vi "数据库访问.vi"() -> ()   [LabVIEW 2018]
uses:
  <vilib>/addons/database/Connection.llb/DB Tools Open Connec (Path).vi
  <vilib>/addons/database/NI_Database_API.lvlib
panel:
  in  "停止":bool
  in  "确定按钮":bool
  out "疫苗数据":T1 {"生产日期" format="%<%Y/%m/%d>T"}
  out "牛奶数据":T2 {"生产日期" format="%<%Y/%m/%d>T"}
  in  "负责人":i32=10003
  in  "牛奶编号":i32=20001
  in  "员工编号":i32=20002
  out "负责人":i32
  out "负责人数据":T3
  out "储运信息":T4 {"记录时间" format="%<%H:%M:%S>T"}
  in  "疫苗编号":i32=10002
  in  "路径":path=path "D:/2019毕业设计/Code/GPData.udl"
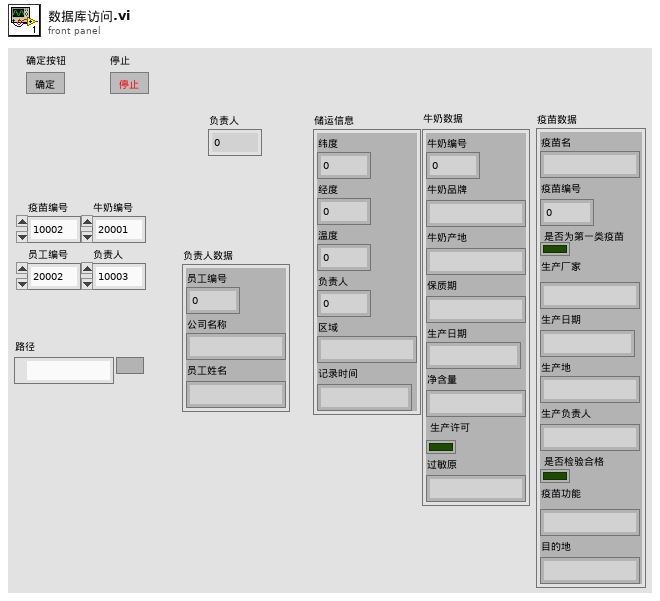
[diagram p1: front panel]
types:
  T1 = typedef "疫苗信息.ctl" = cluster{"疫苗名":string, "疫苗编号":i32, "是否为第一类疫苗":bool, "生产厂家":string, "生产日期":timestamp, "生产地":string, "生产负责人":string, "是否检验合格":bool, "疫苗功能":string, "目的地":string}
  T2 = typedef "牛奶信息.ctl" = cluster{"牛奶编号":i32, "牛奶品牌":string, "牛奶产地":string, "保质期":string, "生产日期":timestamp, "净含量":string, "生产许可":bool, "过敏原":string}
  T3 = typedef "人员信息.ctl" = cluster{"员工编号":i32, "公司名称":string, "员工姓名":string}
  T4 = typedef "储运信息.ctl" = cluster{"纬度":sgl, "经度":sgl, "温度":sgl, "负责人":i32, "区域":string, "记录时间":timestamp}
  T5 = typedef "NI_Database_API.lvlib/Conn ObjectReference.ctl" = refnum<k1>
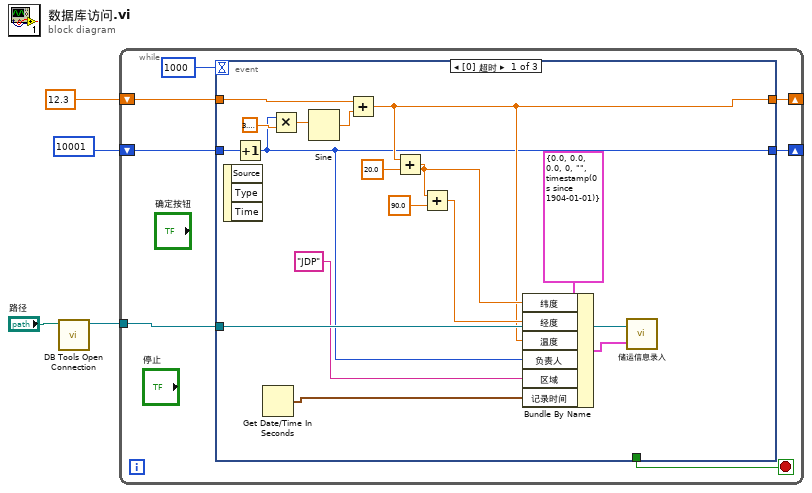
[diagram p0: block diagram]
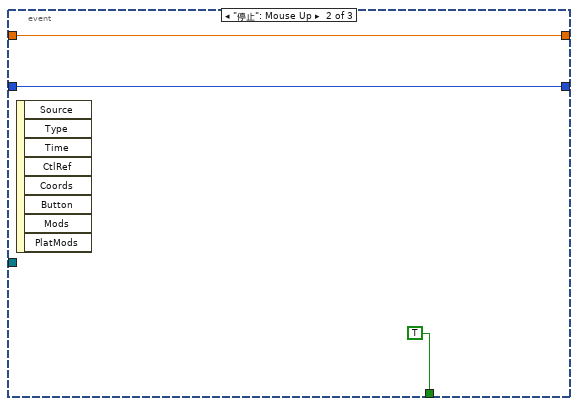
[diagram p2: hidden frame]
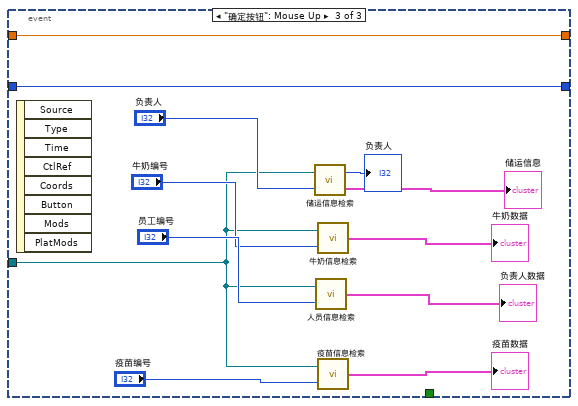
[diagram p3: hidden frame]
diagram:
  n1 = call-poly <vilib>:"DB Tools Open Connection.vi"("connection information"="路径") -> ("connection reference"=w3:T5)  [unwired: 7 in, 1 out]
  n2 = while {
    tunnel: w3 -> [w11]
    shift-right: [w8] -> _
    shift-left: 10001 -> [w7]
    shift-right: [w5] -> _
    shift-left: 12.3 -> [w6]
    stop <- w9 stop-if-true
    n3 = event shown="[0] 超时" {
      selector: _ -> [_ _ _]
      dyn-events: _ -> [_ _ _]
      timeout: 1000 -> [_ _ _]
      tunnel: w11 -> [w27 _ w33]
      tunnel: [_ TRUE _] -> w9
      tunnel: [w16 w28 w32] -> w8
      tunnel: w7 -> [w26 w28 w32]
      tunnel: w6 -> [w25 w29 w31]
      tunnel: [w17 w29 w31] -> w5
      event Timeout {
        n4 = event-data() -> ()  [unwired: 1 in, 3 out]
        n5 = Increment(x=w26) -> (x+1=w16:i32)
        n6 = Get Date/Time In Seconds() -> (seconds since 1Jan1904=w12:timestamp)
        n7 = Multiply(x=w16, y=3.141592653589793) -> (x*y=w23:dbl)
        n8 = Sine(x=w23) -> (sin(x)=w22:dbl)
        n9 = Add(x=w25, y=w22) -> (x+y=w17:dbl)
        n10 = Add(x=w17, y=20.0) -> (x+y=w19:dbl)
        n11 = Add(x=w19, y=90.0) -> (x+y=w18:dbl)
        n12 = Bundle By Name(cluster=T4 {"纬度"=0.0, "经度"=0.0, "温度"=0.0, "负责人"=0, "区域"="", "记录时间"=timestamp(0 s since 1904-01-01)} ("储运信息 2"), "纬度"=w19, "经度"=w18, "温度"=w17, "负责人"=w16, "区域"="JDP", "记录时间"=w12) -> (w13:T4)
        n13 = call "储运信息录入.vi"("簇"=w13, "connection reference"=w27) -> ()  [unwired: 1 out]
      }
      event "停止": Mouse Up {
        n14 = event-data() -> ()  [unwired: 1 in, 8 out]
      }
      event "确定按钮": Mouse Up {
        n15 = event-data() -> ()  [unwired: 1 in, 8 out]
        n16 = call "储运信息检索.vi"("负责人"="负责人", "connection reference"=w33) -> ("储运信息"=→"储运信息":T4, "负责人"=→"负责人":i32)
        n17 = call "人员信息检索.vi"("工作人员编号"="员工编号", "connection reference"=w33) -> ("负责人数据"=→"负责人数据":T3)
        n18 = call "牛奶信息检索.vi"("牛奶编号"="牛奶编号", "connection reference"=w33) -> ("牛奶数据"=→"牛奶数据":T2)
        n19 = call "疫苗信息检索.vi"("疫苗编号"="疫苗编号", "connection reference"=w33) -> ("疫苗数据"=→"疫苗数据":T1)
      }
    }
  }
